vi "Open Example Finder.vi"(1 "Parameters to pass":string) -> ()   [LabVIEW 2015, in "QControl Creation Wizard.lvclass"]
uses:
  QControl Creation Wizard.lvclass
  <helpdir>/_exfinder.llb/NI Shared Directory Type.ctl
  <resource>/dialog/lvconfig.llb/LV Config Read String.vi
panel:
  in  "launch message":string="Launching the NI Example Finder..."
  in  "Get Licensed Version":T1(ring)
  in  "PathToUNIXPathString.vi":refnum<vi>
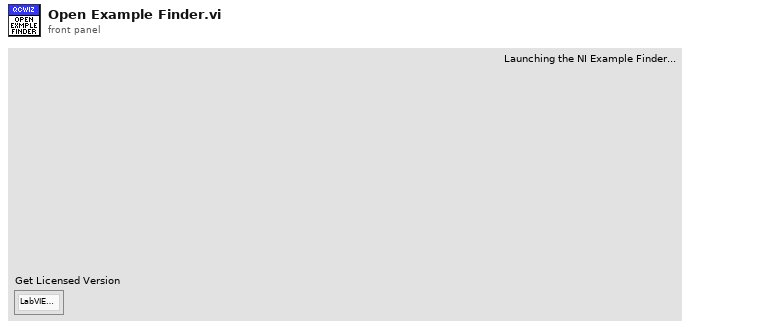
[diagram p1: front panel]
types:
  T1 = enum32{"LabVIEW Pro", "LabVIEW Full", "LabVIEW Base", "LabVIEW Eval", "LabVIEW Student", "LabVIEW Player", "Unlicensed", "LabVIEW Debug Deployment"}
  T2 = typedef "NI Shared Directory Type.ctl" = enum16{"kDefaultSharedDir", "k32bitSharedDir", "k64bitSharedDir"}
  T3 = enum32{"invalid OS target", "Mac OS", "Windows 3.1", "Windows 95/NT", "Solaris 1", "Solaris 2", "HP-UX", "PowerMAX", "Linux", "Irix", "Rhapsody", "BeOS", "AIX", "OSF1", "VxWorks", "PharLap", "Carbon", "RTX", "Windows x64", "Linux x64", "Mac OS X x64"}
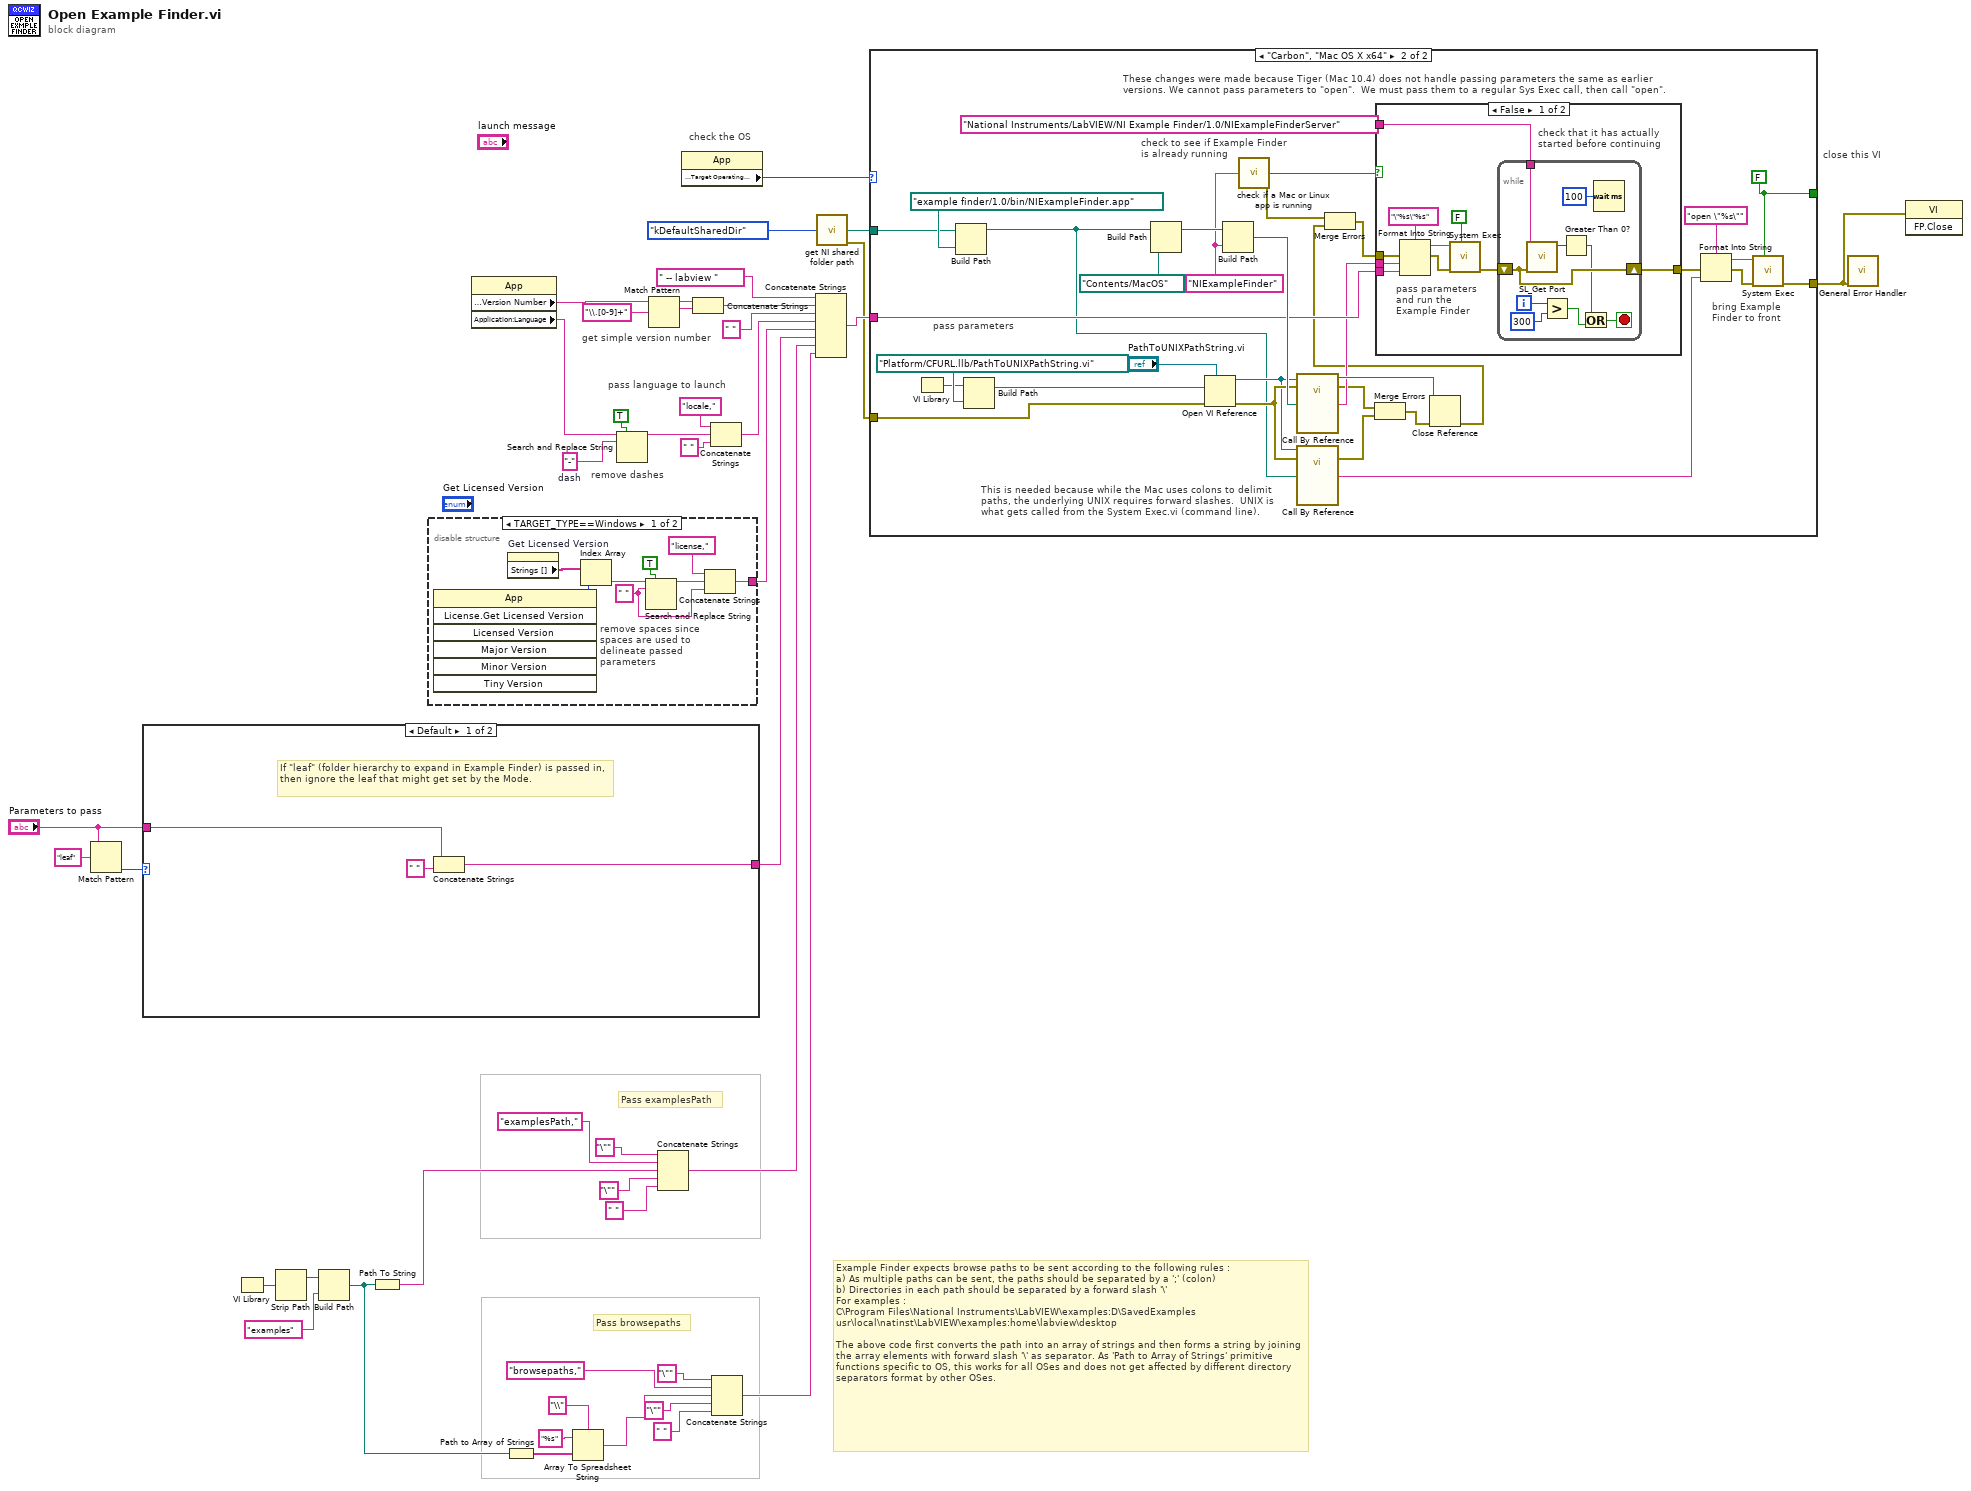
[diagram p0: block diagram]
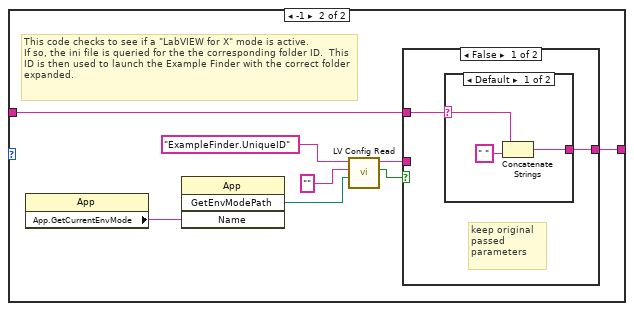
[diagram p2: hidden frame]
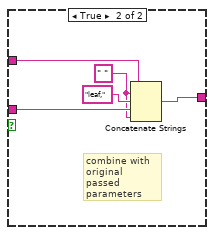
[diagram p4: hidden frame]
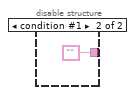
[diagram p5: hidden frame]
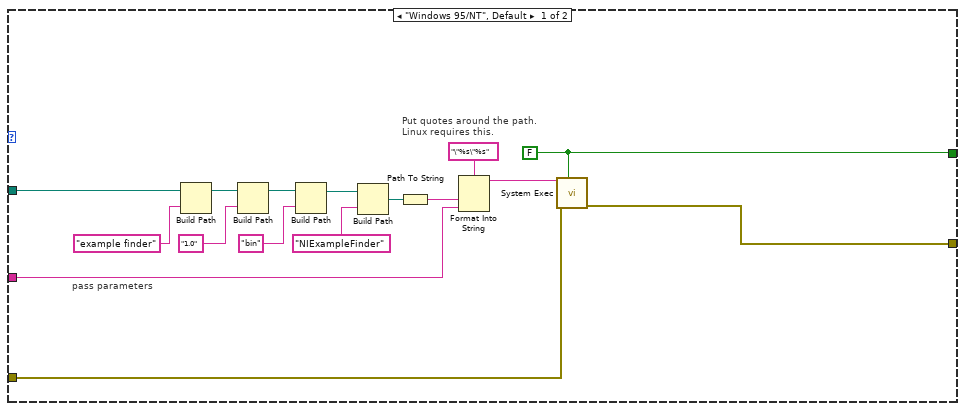
[diagram p6: hidden frame]
diagram:
  w27 = "-"  # dash
  # "Example Finder expects browse paths to be sent according to the following rules :\na) As multiple paths can be sent, the paths should be separated by a ';' (colon)\nb) Directories in each path should be separated by a forward slash '\\' \nFor examples :   \nC\\Program Files\\National Instruments\\LabVIEW\\examples:D\\SavedExamples\nusr\\local\\natinst\\LabVIEW\\examples:home\\labview\\desktop\n\nThe above code first converts the path into an array of strings and then forms a string by joining the array elements with forward slash '\\' as separator. As 'Path to Array of Strings' primitive functions specific to OS, this works for all OSes and does not get affected by different directory separators format by other OSes."
  # "Pass browsepaths"
  # "Pass examplesPath"
  # "remove dashes"
  # "pass language to launch"
  # "close this VI"
  # "get simple version number"
  # "check the OS"
  n1 = Match Pattern(string="Parameters to pass", regular expression="leaf") -> (offset past match=w21:i32)  [unwired: 1 in, 3 out]
  n2 = case shown="Default" w21 {
    tunnel: [w46 w55] -> w24
    tunnel: "Parameters to pass" -> [w47 w54]
    frame Default {
      # "If \"leaf\" (folder hierarchy to expand in Example Finder) is passed in, then ignore the leaf that might get set by the Mode."
      n3 = Concatenate Strings(w47, " " ("string")) -> (w46:string)
    }
    frame -1 {
      # "This code checks to see if a \"LabVIEW for X\" mode is active.  \nIf so, the ini file is queried for the the corresponding folder ID.  This ID is then used to launch the Example Finder with the correct folder expanded."
      n4 = property class="App"() -> ("App.GetCurrentEnvMode"=w48:string)  [unwired: 2 in, 2 out]
      n5 = invoke class="App" method="GetEnvModePath"("Name"=w48) -> ("GetEnvModePathh"=w51:path)  [unwired: 3 in, 3 out]
      n6 = call-poly <resource>:"LV Config Read.vi"("config file path"=w51, "default value"="", "key"="ExampleFinder.UniqueID") -> ("found?"=w50:bool, "value"=w49:string)  [unwired: 2 in, 1 out]
      n7 = case shown="False" w50 {
        tunnel: w49 -> [_ w66]
        tunnel: [w56 w65] -> w55
        tunnel: w54 -> [w57 w64]
        frame False {
          # "keep original passed parameters"
          n8 = case shown="Default" w57 {
            selector: w57 -> [w58 w61]
            tunnel: [w59 w61] -> w56
            frame Default {
              n9 = Concatenate Strings(w58, " " ("string")) -> (w59:string)
            }
            frame "" {
            }
          }
        }
        frame True {
          w62 = " " ("string")
          # "combine with original passed parameters"
          n10 = Concatenate Strings(w64, w62, "leaf," ("string"), w66, w62) -> (w65:string)
        }
      }
    }
  }
  n11 = VI Library() -> (path=w20:path)
  n12 = Strip Path(path=w20) -> (stripped path=w19:path)  [unwired: 1 out]
  n13 = Build Path(base path=w19, name or relative path="examples") -> (appended path=w3:path)
  n14 = Path To String(path=w3) -> (string=w18:string)
  n15 = disable-structure shown="TARGET_TYPE==Windows" {
    disable-tunnel: [w67 ""] -> w33
    frame condition #0 (active) {
      w68 = " " ("search string")
      # "remove spaces since spaces are used to delineate passed parameters"
      n16 = invoke class="App" method="License.Get Licensed Version"() -> ("Get Licensed Version"=w73:T1)  [unwired: 7 in, 6 out]
      n17 = property on="Get Licensed Version" class="Enum (strict)"() -> ("Strings []"=w74:string[])  [unwired: 2 in, 2 out]
      n18 = Index Array(array=w74, index=w73) -> (element=w71:string)
      n19 = Search and Replace String(replace all?=TRUE ("replace all? (F)"), input string=w71, search string=w68) -> (result string=w70:string)  [unwired: 5 in, 3 out]
      n20 = Concatenate Strings("license," ("string"), w70, w68) -> (w67:string)
    }
    frame condition #1 {
    }
  }
  n21 = property class="App"() -> ("Application:Version Number"=w40:string, "Application:Language"=w28:string)  [unwired: 2 in, 2 out]
  n22 = Path to Array of Strings(0:w3) -> (2:w6:string[])  [unwired: 1 out]
  n23 = Array To Spreadsheet String(delimiter (Tab)="\\", array=w6, 3:"%s" ("format string")) -> (spreadsheet string=w2:string)
  n24 = Search and Replace String(replace all?=TRUE ("replace all? (F)"), input string=w28, search string=w27) -> (result string=w29:string)  [unwired: 5 in, 3 out]
  n25 = Match Pattern(string=w40, regular expression="\\.[0-9]+") -> (before substring=w38:string, match substring=w39:string)  [unwired: 1 in, 2 out]
  n26 = Concatenate Strings("\"" ("string"), "examplesPath," ("string"), w18, "\"" ("string"), " " ("string")) -> (w8:string)
  n27 = property class="App"() -> ("Application:Target Operating System"=w43:T3)  [unwired: 2 in, 2 out]
  n28 = Concatenate Strings(w38, w39) -> (w36:string)
  n29 = Concatenate Strings("locale," ("string"), w29, " " ("name or relative path")) -> (w35:string)
  n30 = Concatenate Strings("\"" ("string"), "browsepaths," ("string"), w2, "\"" ("string"), " " ("string")) -> (w7:string)
  n31 = Concatenate Strings(" -- labview " ("name or relative path"), w36, " " ("name or relative path"), w35, w33, w24, w8, w7) -> (w41:string)
  n32 = call <helpdir>:"get NI shared folder path.vi"("NI Shared Directory Type"=NI_Shared_Directory_Type."kDefaultSharedDir") -> ("shared folder path"=w44:path, "error out"=w32:errorcluster)  [unwired: 13 in]
  n33 = case shown="\"Carbon\", \"Mac OS X x64\"" w43 {
    tunnel: [w88 w112] -> w1
    tunnel: w44 -> [w82 w97]
    tunnel: [w78 w104] -> _
    tunnel: w41 -> [w77 w118]
    tunnel: w32 -> [w76 w103]
    frame "Windows 95/NT", Default {
      w78 = FALSE ("wait until completion? (T)")
      # "Put quotes around the path.\nLinux requires this."
      # "pass parameters"
      n34 = Build Path(base path=w82, name or relative path="example finder") -> (appended path=w90:path)
      n35 = Build Path(base path=w90, name or relative path="1.0") -> (appended path=w86:path)
      n36 = Build Path(base path=w86, name or relative path="bin") -> (appended path=w85:path)
      n37 = Build Path(base path=w85, name or relative path="NIExampleFinder") -> (appended path=w83:path)
      n38 = Path To String(path=w83) -> (string=w81:string)
      n39 = Format Into String(format string="\"%s\"%s", w81, w77) -> (resulting string=w80:string)  [unwired: 2 in, 1 out]
      n40 = call <vilib>:"System Exec.vi"("wait until completion? (T)"=w78, "error in (no error)"=w76, "command line"=w80) -> ("error out"=w88:errorcluster)  [unwired: 5 in, 3 out]
    }
    frame "Carbon", "Mac OS X x64" {
      w104 = FALSE ("wait until completion? (T)")
      w102 = "NIExampleFinder" ("name or relative path")
      # "These changes were made because Tiger (Mac 10.4) does not handle passing parameters the same as earlier versions. We cannot pass parameters to \"open\".  We must pass them to a regular Sys Exec call, then call \"open\"."
      # "bring Example Finder to front"
      # "check to see if Example Finder is already running"
      # "This is needed because while the Mac uses colons to delimit paths, the underlying UNIX requires forward slashes.  UNIX is what gets called from the System Exec.vi (command line)."
      # "pass parameters"
      n41 = VI Library() -> (path=w94:path)
      n42 = Build Path(base path=w97, name or relative path=path "example finder/1.0/bin/NIExampleFinder.app" ("appended path")) -> (appended path=w93:path)
      n43 = Build Path(base path=w94, name or relative path=path "Platform/CFURL.llb/PathToUNIXPathString.vi" ("appended path")) -> (appended path=w122:path)
      n44 = Build Path(base path=w93, name or relative path=path "Contents/MacOS" ("appended path")) -> (appended path=w120:path)
      n45 = Open VI Reference(type specifier VI Refnum (for type only)="PathToUNIXPathString.vi", vi path=w122, error in (no error)=w103) -> (vi reference=w109:refnum<vi>, error out=w110:errorcluster)  [unwired: 3 in]
      n46 = Build Path(base path=w120, name or relative path=w102) -> (appended path=w119:path)
      n47 = call <helpdir>:"check if a Mac or Linux app is running.vi"("Mac or Linux app to check"=w102) -> ("app is running"=w101:bool, "error out"=w100:errorcluster)  [unwired: 13 in]
      n48 = call-by-ref "?"(reference=w109, error in=w110, "LV Path"=w119) -> (reference out=w123:refnum<vi>, error out=w108:errorcluster, "UNIX Path"=w111:string)  [unwired: 1 in, 1 out]
      n49 = call-by-ref "?"(reference=w109, error in=w110, "LV Path"=w93) -> (error out=w107:errorcluster, "UNIX Path"=w105:string)  [unwired: 1 in, 2 out]
      n50 = Merge Errors(w108, w107) -> (w106:errorcluster)
      n51 = Close Reference(reference=w123, error in (no error)=w106) -> (error out=w99:errorcluster)
      n52 = Merge Errors(w100, w99) -> (w117:errorcluster)
      n53 = case shown="False" w101 {
        tunnel: w111 -> [w133 _]
        tunnel: w118 -> [w132 _]
        tunnel: w117 -> [w128 w143]
        tunnel: [w125 w143] -> w113
        tunnel: "National Instruments/LabVIEW/NI Example Finder/1.0/NIExampleFinderServer" ("service name") -> [w124 _]
        frame False {
          # "check that it has actually started before continuing"
          # "pass parameters and run the Example Finder"
          n54 = Format Into String(format string="\"%s\"%s", error in=w128, w133, w132) -> (resulting string=w129:string, error out=w127:errorcluster)  [unwired: 1 in]
          n55 = call <vilib>:"System Exec.vi"("wait until completion? (T)"=FALSE, "error in (no error)"=w127, "command line"=w129) -> ("error out"=w126:errorcluster)  [unwired: 5 in, 3 out]
          n56 = while {
            shift-right: [w137] -> w125
            shift-left: w126 -> [w137]
            tunnel: w124 -> [w134]
            i -> [w140]
            stop <- w142 stop-if-true
            n57 = call <vilib>:"SL_Get Port.vi"("error in (no error)"=w137, "service name"=w134) -> ("port"=w136:u16)  [unwired: 8 in, 1 out]
            n58 = Greater?(x=w140, y=300) -> (0:w139:bool)
            n59 = Greater Than 0?(x=w136) -> (x > 0?=w135:bool)
            n60 = Or(x=w135, y=w139) -> (x .or. y?=w142:bool)
            n61 = Wait (ms)(milliseconds to wait=u32 100) -> ()  [unwired: 1 out]
          }
        }
        frame True {
          # "Example Finder is already running"
        }
      }
      n62 = Format Into String(format string="open \"%s\"", error in=w113, w105) -> (resulting string=w115:string, error out=w114:errorcluster)  [unwired: 1 in]
      n63 = call <vilib>:"System Exec.vi"("wait until completion? (T)"=w104, "error in (no error)"=w114, "command line"=w115) -> ("error out"=w112:errorcluster)  [unwired: 5 in, 3 out]
    }
  }
  n64 = call <vilib>:"General Error Handler.vi"("error in (no error)"=w1) -> ()  [unwired: 10 in, 5 out]
  n65 = invoke class="VI" method="FP.Close"(error in=w1) -> ()  [unwired: 2 in, 3 out]
